vi "RT Driver VI.vi"(7 "Operation":T1, 11 "Device Reference in":T2 format="%.0x") -> (0 "Error Code":i32)   [LabVIEW 2016, in "FPGA RM Test Client Engine.lvlib"]
uses:
  FPGA RM Test Client Engine.lvlib
  <vilib>/NI Veristand/Custom Device API/Custom Device Item Ref.ctl
  <vilib>/NI Veristand/Custom Device API/Hardware Interface Driver VI Operation.ctl
  Shared/Compiled.Settings.ctl
  RTStateVariables.ctl
  <vilib>/NI/NIVS Inline Async API/_VS Inline Async API/VS Inline Async API/VS Inline Async API.lvclass
  <vilib>/NI/NIVS Inline Async API/_VS Inline Async API/VS Inline Async API/VS Inline Async API.lvclass/VS Inline Async API.ctl
  <vilib>/NI/NIVS Inline Async API/_Data Access Engine/Data Access Engine/Data Access Engine.lvclass/Data Access Engine.ctl
  <vilib>/NI/NIVS Inline Async API/_Data Access Engine/Access Type Classes/Write/Write.lvclass/Write.ctl
  <vilib>/NI/NIVS Inline Async API/_Data Access Engine/Access Type Classes/ReadWrite/ReadWrite.lvclass/ReadWrite.ctl
  <vilib>/NI/NIVS Inline Async API/_Data Access Engine/Access Type Classes/Read/Read.lvclass/Read.ctl
  <vilib>/NI/NIVS Inline Async API/_Data Access Engine/Data Access Engine/Methods/Data.Engine.Read Data from HW.vi
  <vilib>/NI/NIVS Inline Async API/_VS Inline Async API/Error Handling Process/SubVIs/Error.GetError.vi
  <vilib>/NI/NIVS Inline Async API/_Data Access Engine/Data Access Engine/Methods/Data.Engine.Write Data to HW.vi
  <vilib>/NI/NIVS Inline Async API/_Data Access Engine/Access Type Classes/ReadWrite/ReadWrite.EngineData.vi
  <vilib>/NI/NIVS Inline Async API/_Data Access Engine/Access Type Classes/Write/Write.EngineData.vi
  <vilib>/NI/NIVS Inline Async API/_Data Access Engine/Access Type Classes/Read/Read.EngineData.vi
  <vilib>/NI Veristand/Custom Device API/NI VeriStand - Get Channel Value by Data Reference.vi
  <vilib>/NI Veristand/Custom Device API/NI VeriStand - Set Channel Value by Data Reference.vi
  <vilib>/NI Veristand/Custom Device API/NI VeriStand - Get Channel Values by Block Data Reference.vi
  Shared/Constants.vi
  <vilib>/NI Veristand/Custom Device API/Get Item Property (Variant).vi
  <vilib>/NI Veristand/Custom Device API/Global Data Refs.vi
  <vilib>/NI VeriStand/Custom Device API/Custom Device API.lvlib
  <vilib>/NI VeriStand/Custom Device Tools/Custom Device Utility Library/Custom Device Utility Library.lvlib
  Shared/FPGA RM Test Client Shared.lvlib
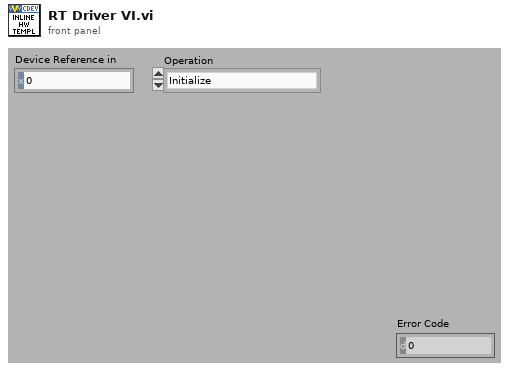
[diagram p1: front panel]
types:
  T1 = typedef "Custom Device API.lvlib/Hardware Interface Driver VI Operation.ctl" = enum16{"Initialize", "Start", "Read Data from HW", "Write Data to HW", "Close"}
  T2 = typedef "Custom Device API.lvlib/Custom Device Item Ref.ctl" = u64
  T3 = typedef "FPGA RM Test Client Engine.lvlib/RTStateVariables.ctl" = cluster{"Async":refnum<class "VS Inline Async API.lvclass">, "Settings":T4}
  T4 = typedef "FPGA RM Test Client Shared.lvlib/Compiled.Settings.ctl" = cluster{"Name":string}
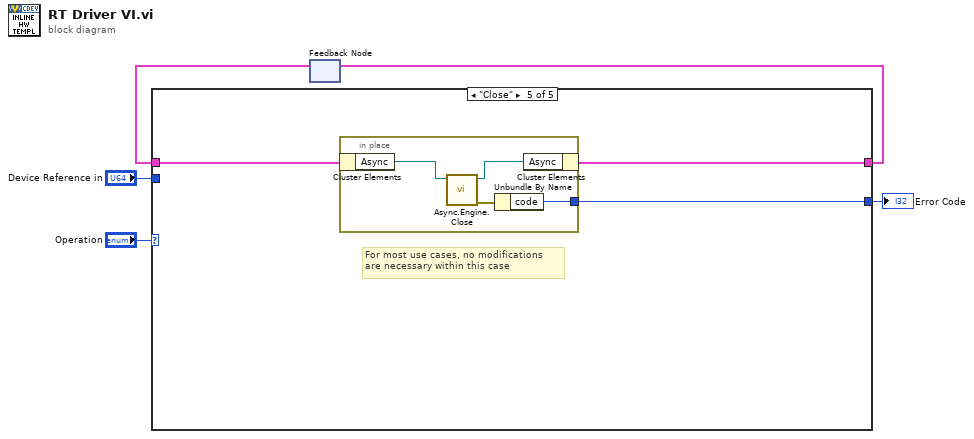
[diagram p0: block diagram]
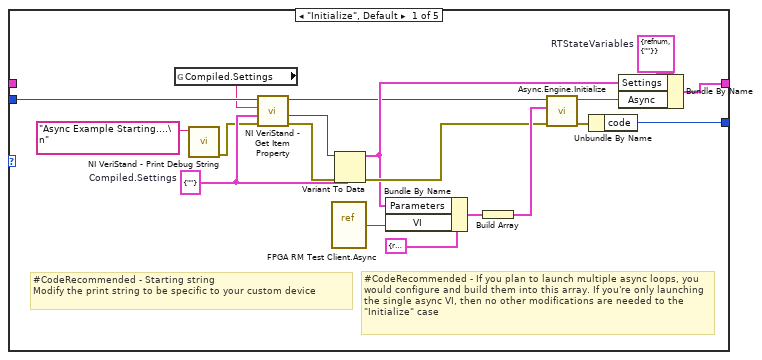
[diagram p2: hidden frame]
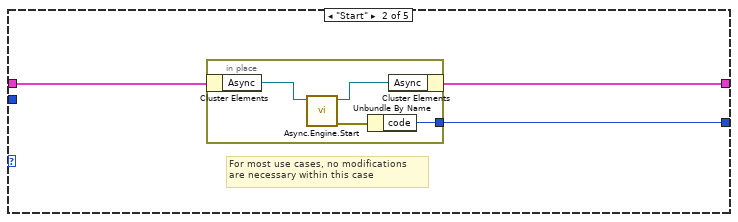
[diagram p3: hidden frame]
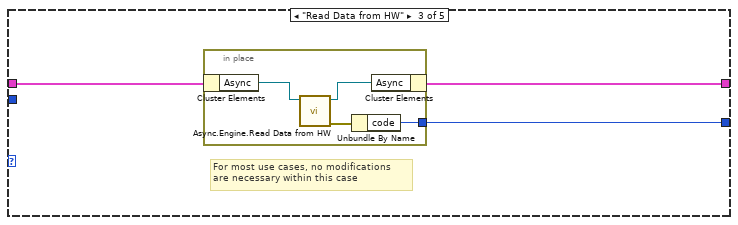
[diagram p4: hidden frame]
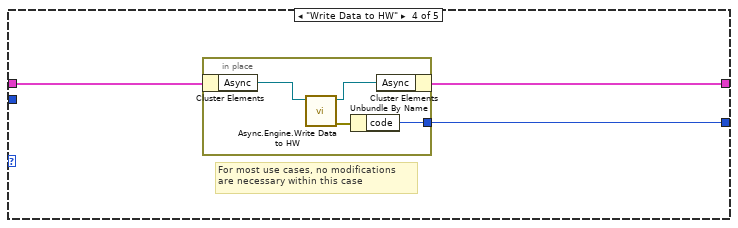
[diagram p5: hidden frame]
diagram:
  n1 = feedback #1() -> (w3:T3)  [unwired: 1 out]
  n2 = case shown="\"Close\"" "Operation" {
    tunnel: [w22 w26 w32 w39 w47] -> w4
    tunnel: w3 -> [_ w27 w34 w40 w48]
    tunnel: "Device Reference in" -> [w19 _ _ _ _]
    tunnel: [w24 w25 w33 w41 w46] -> w1
    frame "Initialize", Default {
      w13 = T3 {"Async"=refnum, "Settings"={"Name"=""}}  # RTStateVariables
      w14 = T4 {"Name"=""}  # Compiled.Settings
      # "#CodeRecommended - Starting string\nModify the print string to be specific to your custom device"
      # "#CodeRecommended - If you plan to launch multiple async loops, you would configure and build them into this array. If you're only launching the single async VI, then no other modifications are needed to the \"Initialize\" case"
      n3 = global read "Constants.vi" "Compiled.Settings"() -> (w16:string)
      n4 = call <vilib>:"NI VeriStand - Print Debug String.vi"("Message"="Async Example Starting....\n") -> ("error out"=w8:errorcluster)  [unwired: 10 in]
      n5 = call-poly <vilib>:"NI VeriStand - Get Item Property.vi"("error in (no error)"=w8, "Default Value"=w14, "Property Name"=w16, "Item Ref in"=w19) -> ("error out"=w18:errorcluster, "Value"=w17:variant, "Item Ref out"=w9:T2)  [unwired: 4 in, 1 out]
      n6 = vi-ref "FPGA RM Test Client.Async.vi"() -> (w6:refnum<vi>)
      n7 = Variant To Data(error in=w18, type=w14, Variant=w17) -> (data=w10:T4, error out=w11:errorcluster)
      n8 = Bundle By Name(cluster=cluster{"VI":refnum<vi>, "Parameters":variant} {"VI"=refnum, "Parameters"=variant} ("Process"), "Parameters"=w10, "VI"=w6) -> (w20:cluster{"VI":refnum<vi>, "Parameters":variant})
      n9 = Build Array(w20) -> (w12:cluster{"VI":refnum<vi>, "Parameters":variant}[])
      n10 = call <vilib>:"Async.Engine.Initialize.vi"("error in (no error)"=w11, "Processes"=w12, "Custom Device Ref"=w9) -> ("error out"=w15:errorcluster, "Async"=w23:refnum<class "VS Inline Async API.lvclass">)  [unwired: 7 in]
      n11 = Unbundle By Name(w15) -> ("code"=w24:i32)
      n12 = Bundle By Name(cluster=w13, "Settings"=w10, "Async"=w23) -> (w22:T3)
    }
    frame "Start" {
      # "For most use cases, no modifications \nare necessary within this case"
      n13 = in-place {
        in-place-border: [w28] -> w25
        n14 = in-place-cluster #2(w27) -> ("Async"=w31:refnum<class "VS Inline Async API.lvclass">)
        n15 = call <vilib>:"Async.Engine.Start.vi"("VS Inline Async API in"=w31) -> ("error out"=w29:errorcluster, "VS Inline Async API out"=w30:refnum<class "VS Inline Async API.lvclass">)  [unwired: 9 in]
        n16 = Unbundle By Name(w29) -> ("code"=w28:i32)
        n17 = in-place-cluster #2("Async"=w30) -> (w26:T3)
      }
    }
    frame "Read Data from HW" {
      # "For most use cases, no modifications \nare necessary within this case"
      n18 = in-place {
        in-place-border: [w36] -> w33
        n19 = in-place-cluster #3(w34) -> ("Async"=w38:refnum<class "VS Inline Async API.lvclass">)
        n20 = call <vilib>:"Async.Engine.Read Data from HW.vi"("Async in"=w38) -> ("error out"=w35:errorcluster, "Async out"=w37:refnum<class "VS Inline Async API.lvclass">)  [unwired: 9 in]
        n21 = Unbundle By Name(w35) -> ("code"=w36:i32)
        n22 = in-place-cluster #3("Async"=w37) -> (w32:T3)
      }
    }
    frame "Write Data to HW" {
      # "For most use cases, no modifications \nare necessary within this case"
      n23 = in-place {
        in-place-border: [w45] -> w41
        n24 = in-place-cluster #4(w40) -> ("Async"=w43:refnum<class "VS Inline Async API.lvclass">)
        n25 = call <vilib>:"Async.Engine.Write Data to HW.vi"("VS Inline Async API in"=w43) -> ("error out"=w44:errorcluster, "VS Inline Async API out"=w42:refnum<class "VS Inline Async API.lvclass">)  [unwired: 9 in]
        n26 = Unbundle By Name(w44) -> ("code"=w45:i32)
        n27 = in-place-cluster #4("Async"=w42) -> (w39:T3)
      }
    }
    frame "Close" {
      # "For most use cases, no modifications \nare necessary within this case"
      n28 = in-place {
        in-place-border: [w50] -> w46
        n29 = in-place-cluster #5(w48) -> ("Async"=w52:refnum<class "VS Inline Async API.lvclass">)
        n30 = call <vilib>:"Async.Engine.Close.vi"("Async in"=w52) -> ("error out"=w49:errorcluster, "Async out"=w51:refnum<class "VS Inline Async API.lvclass">)  [unwired: 9 in]
        n31 = Unbundle By Name(w49) -> ("code"=w50:i32)
        n32 = in-place-cluster #5("Async"=w51) -> (w47:T3)
      }
    }
  }
  "Error Code" <- w1
  n33 = feedback-in #1(w4) -> ()
